vi "ControlRoom-RT.vi"() -> ()   [LabVIEW 2016]
uses:
  <vilib>/FPGAPlugInAG/cRIO-9074/niLvFpga_Open_cRIO-9074.vi
  <vilib>/Utility/error.llb/Error Cluster From Error Code.vi
  <vilib>/rvi/errors/niLvFpgaAdjustHostInterfaceError.vi
  <vilib>/rvi/interface/nirviOpenFPGA/nirviOpenFPGA.xnode
  FPGA Bitfiles/ControlRm-2016_FPGATarget_ControlRoom-FPGA_fnicreUWpIg.lvbitx
  ControlRoom-FPGA.vi
  <vilib>/rvi/interface/nirviReadWriteControl/nirviReadWriteControl.xnode
  NiFpgaLv.dll
panel:
  out "Le Sup":fxp<+/-,26,5> format="%_3g"
  out "Le Ind":fxp<+/-,26,5> format="%_3g"
  out "Le chain":fxp<+/-,26,5> format="%_3g"
  out "Le column":fxp<+/-,26,5> format="%_3g"
  out "He column":fxp<+/-,26,5> format="%_3g"
  out "He chain":fxp<+/-,26,5> format="%_3g"
  out "He Ind":fxp<+/-,26,5> format="%_3g"
  out "He Sup":fxp<+/-,26,5> format="%_3g"
  out "Grid":fxp<+/-,26,5> format="%_3g"
  out "Corona":fxp<+/-,26,5> format="%_3g"
  out "Terminal voltage":fxp<+/-,26,5> format="%_3g"
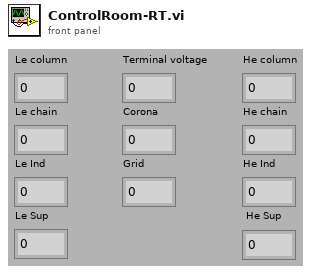
[diagram p1: front panel]
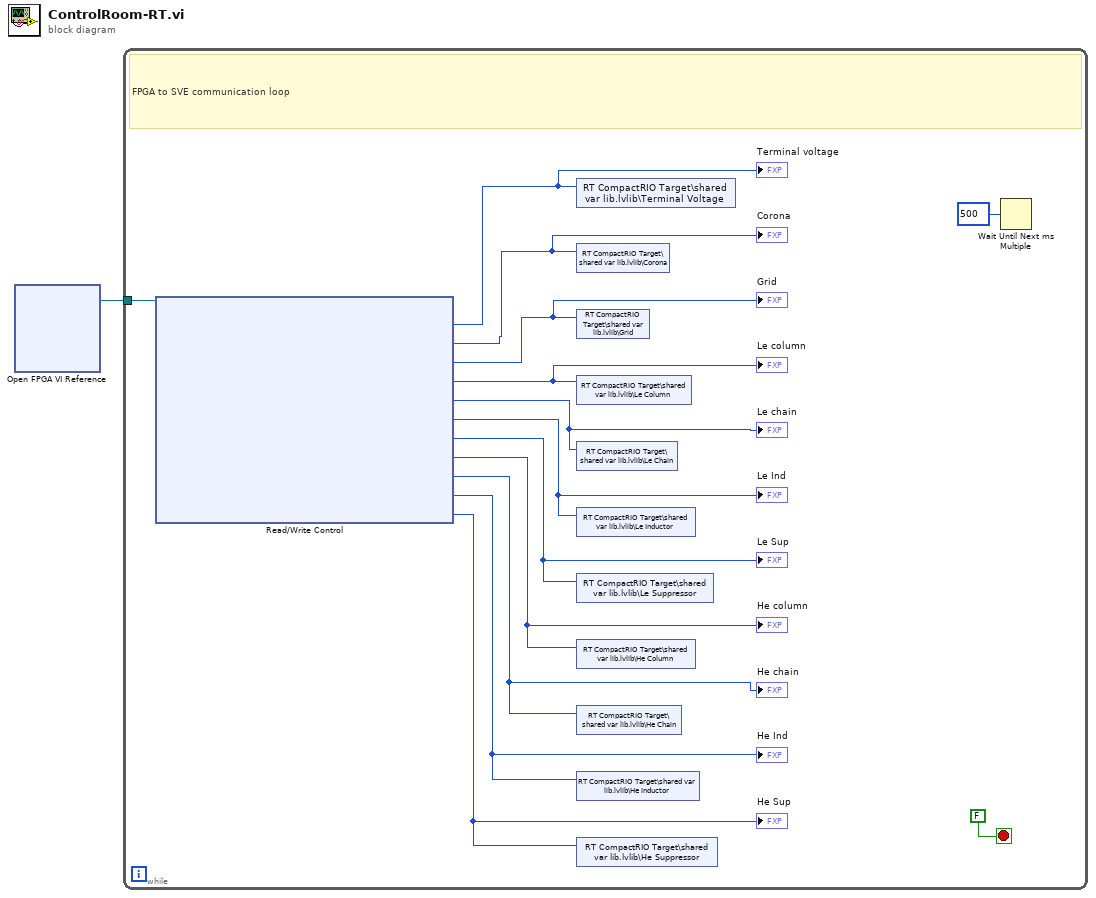
[diagram p0: block diagram]
diagram:
  n1 = xnode "Open FPGA VI Reference"() -> ("FPGA VI Reference Out"=w1:refnum<k20>)  [unwired: 2 in, 1 out]
  n2 = while {
    tunnel: w1 -> [w13]
    stop <- FALSE stop-if-true
    # "FPGA to SVE communication loop"
    n3 = xnode "Read/Write Control"("FPGA VI Reference In"=w13) -> ("Terminal Readbacks.GVM Voltage"=w12:i16, "Terminal Readbacks.Corona Probe Current"=w11:i16, "Terminal Readbacks.Grid Voltage"=w10:i16, "LE Readbacks.Column Current"=w9:i16, "LE Readbacks.Chain Current"=w8:i16, "LE Readbacks.Inductor"=w7:i16, "LE Readbacks.Suppressor"=w6:i16, "HE Readbacks.Column Current"=w5:i16, "HE Readbacks.Chain Current"=w4:i16, "HE Readbacks.Inductor"=w3:i16, "HE Readbacks.Suppressor"=w2:i16)  [unwired: 1 in, 2 out]
    "Terminal voltage" <- w12
    "Corona" <- w11
    "Grid" <- w10
    "He Sup" <- w2
    "He Ind" <- w3
    "He chain" <- w4
    "He column" <- w5
    "Le Sup" <- w6
    "Le Ind" <- w7
    "Le chain" <- w8
    "Le column" <- w9
    n4 = shared-variable "RT CompactRIO Target\\shared var lib.lvlib\\Terminal Voltage"(w12) -> ()  [unwired: 1 in, 1 out]
    n5 = shared-variable "RT CompactRIO Target\\shared var lib.lvlib\\Corona"(w11) -> ()  [unwired: 1 in, 1 out]
    n6 = shared-variable "RT CompactRIO Target\\shared var lib.lvlib\\Grid"(w10) -> ()  [unwired: 1 in, 1 out]
    n7 = shared-variable "RT CompactRIO Target\\shared var lib.lvlib\\Le Column"(w9) -> ()  [unwired: 1 in, 1 out]
    n8 = shared-variable "RT CompactRIO Target\\shared var lib.lvlib\\Le Chain"(w8) -> ()  [unwired: 1 in, 1 out]
    n9 = shared-variable "RT CompactRIO Target\\shared var lib.lvlib\\Le Inductor"(w7) -> ()  [unwired: 1 in, 1 out]
    n10 = shared-variable "RT CompactRIO Target\\shared var lib.lvlib\\Le Suppressor"(w6) -> ()  [unwired: 1 in, 1 out]
    n11 = shared-variable "RT CompactRIO Target\\shared var lib.lvlib\\He Column"(w5) -> ()  [unwired: 1 in, 1 out]
    n12 = shared-variable "RT CompactRIO Target\\shared var lib.lvlib\\He Chain"(w4) -> ()  [unwired: 1 in, 1 out]
    n13 = shared-variable "RT CompactRIO Target\\shared var lib.lvlib\\He Inductor"(w3) -> ()  [unwired: 1 in, 1 out]
    n14 = shared-variable "RT CompactRIO Target\\shared var lib.lvlib\\He Suppressor"(w2) -> ()  [unwired: 1 in, 1 out]
    n15 = Wait Until Next ms Multiple(millisecond multiple=u32 500) -> ()  [unwired: 1 out]
  }
